vi "main.vi"() -> ()   [LabVIEW 2015]
panel:
  out "?":T1(plugin-control)
  in  "Reference":string
  out "Test PASS":bool
  out "Temp De Test (en S)":dbl format="%#_3g"
  in  "Numeo Serie":string
  out "Total Carte":dbl caption="Total  Carte :"
  out "Carte Fail":dbl caption="Carte Fail :"
  out "Carte Pass":dbl caption="Carte Pass :"
  # "Carte à tester"
  # "Poste Vision"
  # "copyright © www.corail-technologie.com"
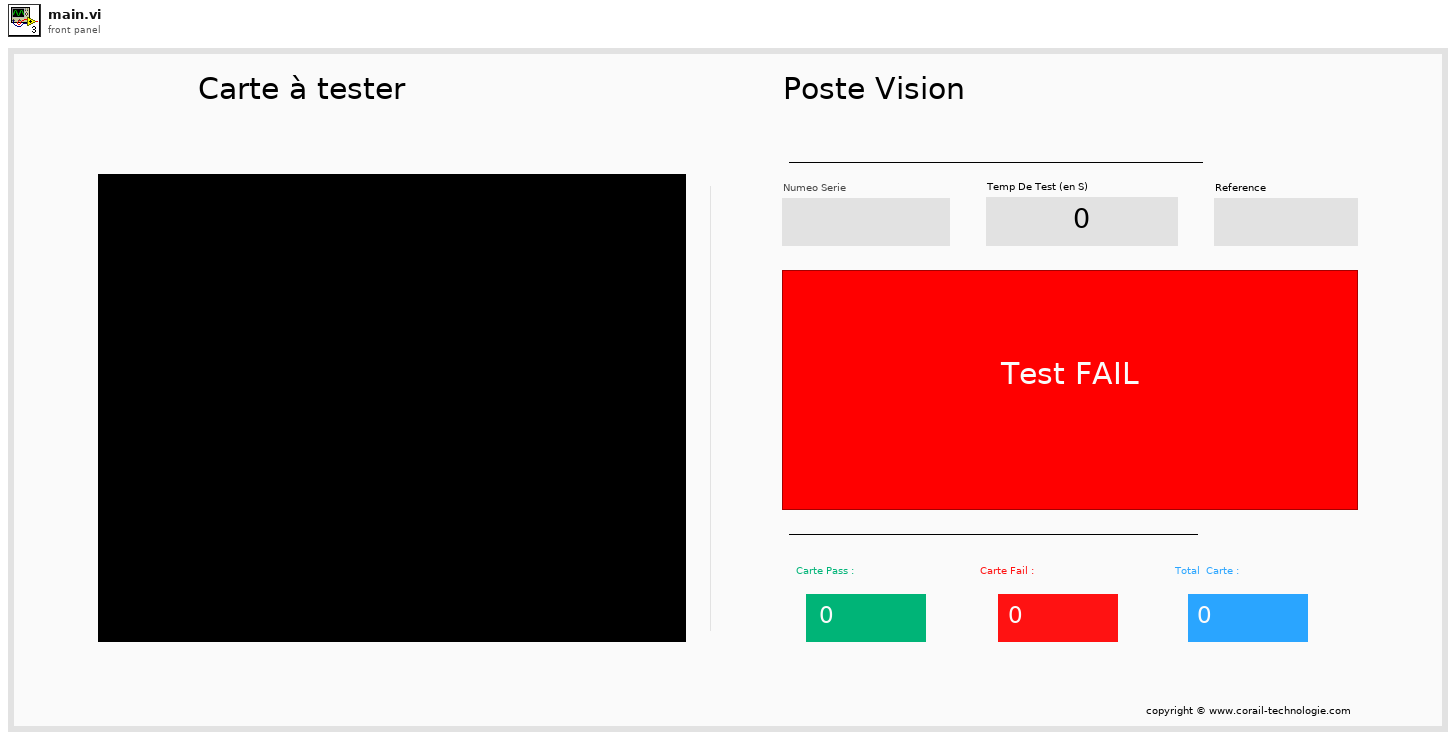
[diagram p1: front panel]
types:
  T1 = typedef "IMAQ Image.ctl" = refnum<image>
  T2 = typedef "VBAIInterface.ctl" = refnum<k21>
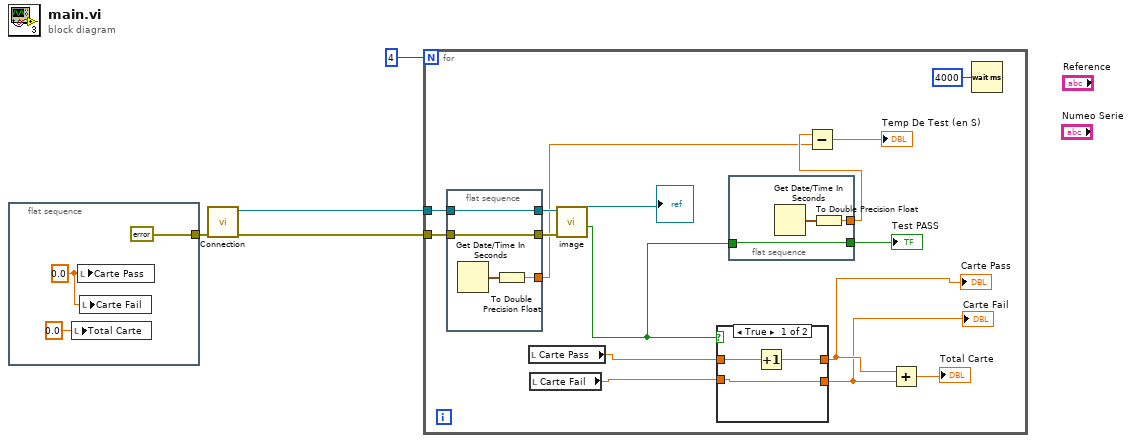
[diagram p0: block diagram]
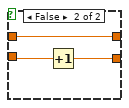
[diagram p2: hidden frame]
diagram:
  n1 = flat-sequence {
    tunnel: [errorcluster {"status"=FALSE, "code"=0, "source"=""} ("error in")] -> w2
    frame #0 {
      w5 = 0.0 ("Carte Pass")
      n2 = local write "Total Carte"(0.0 ("Total Carte")) -> ()
      n3 = local write "Carte Pass"(w5) -> ()
      n4 = local write "Carte Fail"(w5) -> ()
    }
  }
  n5 = call "Connection.vi"("error in"=w2) -> ("error out"=w1:errorcluster, "Session Out"=w4:T2)  [unwired: 9 in]
  n6 = for {
    N: 4 -> [_]
    tunnel: w1 -> [w14]
    tunnel: w4 -> [w16]
    n7 = flat-sequence {
      tunnel: [w30] -> w17
      tunnel: w16 -> [w30]
      tunnel: [w29] -> w15
      tunnel: w14 -> [w29]
      tunnel: [w27] -> w12
      frame #0 {
        n8 = Get Date/Time In Seconds() -> (seconds since 1Jan1904=w28:timestamp)
        n9 = To Double Precision Float(number=w28) -> (double precision float=w27:dbl)
      }
    }
    n10 = local read "Carte Pass"() -> (w22:dbl)
    n11 = local read "Carte Fail"() -> (w21:dbl)
    n12 = call "image.vi"("error in"=w15, "Session In"=w17) -> ("Inspection Status"=w10:bool, "Image"=→"?":T1)  [unwired: 7 in, 1 out]
    n13 = case shown="True" w10 {
      tunnel: w22 -> [w33 w35]
      tunnel: [w32 w35] -> w20
      tunnel: [w31 w36] -> w19
      tunnel: w21 -> [w31 w34]
      frame True {
        n14 = Increment(x=w33) -> (x+1=w32:dbl)
      }
      frame False {
        n15 = Increment(x=w34) -> (x+1=w36:dbl)
      }
    }
    "Carte Pass" <- w20
    "Carte Fail" <- w19
    n16 = flat-sequence {
      tunnel: [w25] -> w13
      tunnel: w10 -> [w24]
      tunnel: [w24] -> w9
      frame #0 {
        n17 = Get Date/Time In Seconds() -> (seconds since 1Jan1904=w26:timestamp)
        n18 = To Double Precision Float(number=w26) -> (double precision float=w25:dbl)
      }
    }
    n19 = Subtract(x=w13, y=w12) -> (x-y=→"Temp De Test (en S)":dbl)
    n20 = Add(x=w20, y=w19) -> (x+y=→"Total Carte":dbl)
    n21 = Wait (ms)(milliseconds to wait=u32 4000) -> ()  [unwired: 1 out]
    "Test PASS" <- w9
  }
